vi "_wmg_readItems.vi"(2 "input_p":i32[](array[numeric]), 3 "input":string[](array[string]), 4 "input_sp":string[](array[string])) -> (0 "output_p":i32[](array[numeric]), 1 "output_sp":string[](array[string]))   [LabVIEW 2011]
panel:
  out "数组":string[](array[string])
  in  "列表框":i32(listbox)
  out "数组 2":i32[](array[numeric])
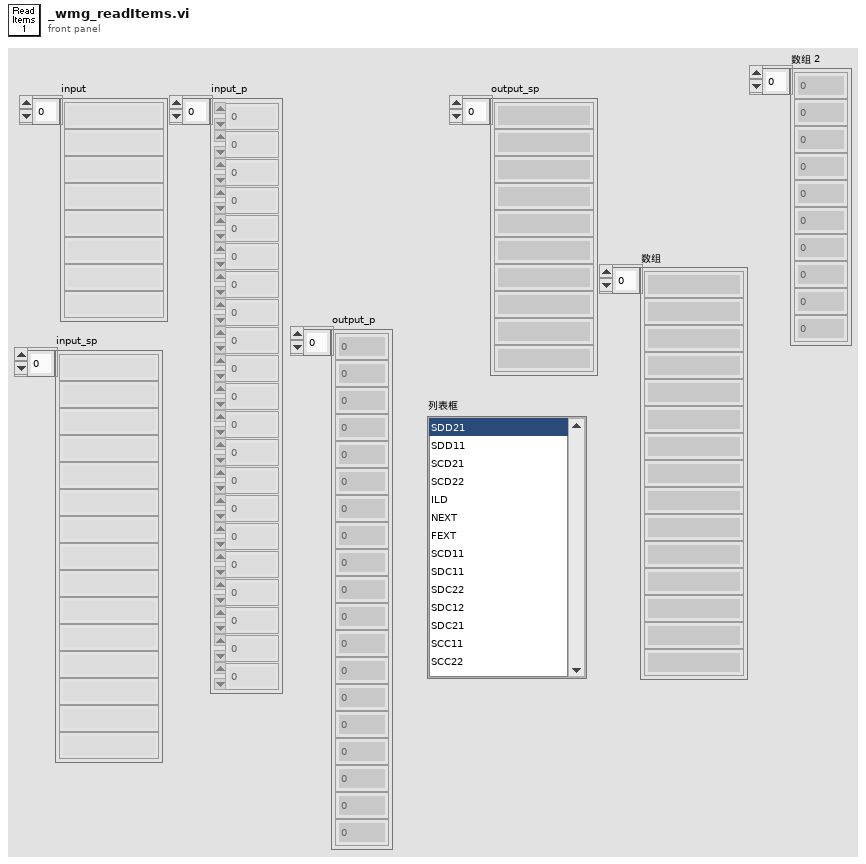
[diagram p1: front panel]
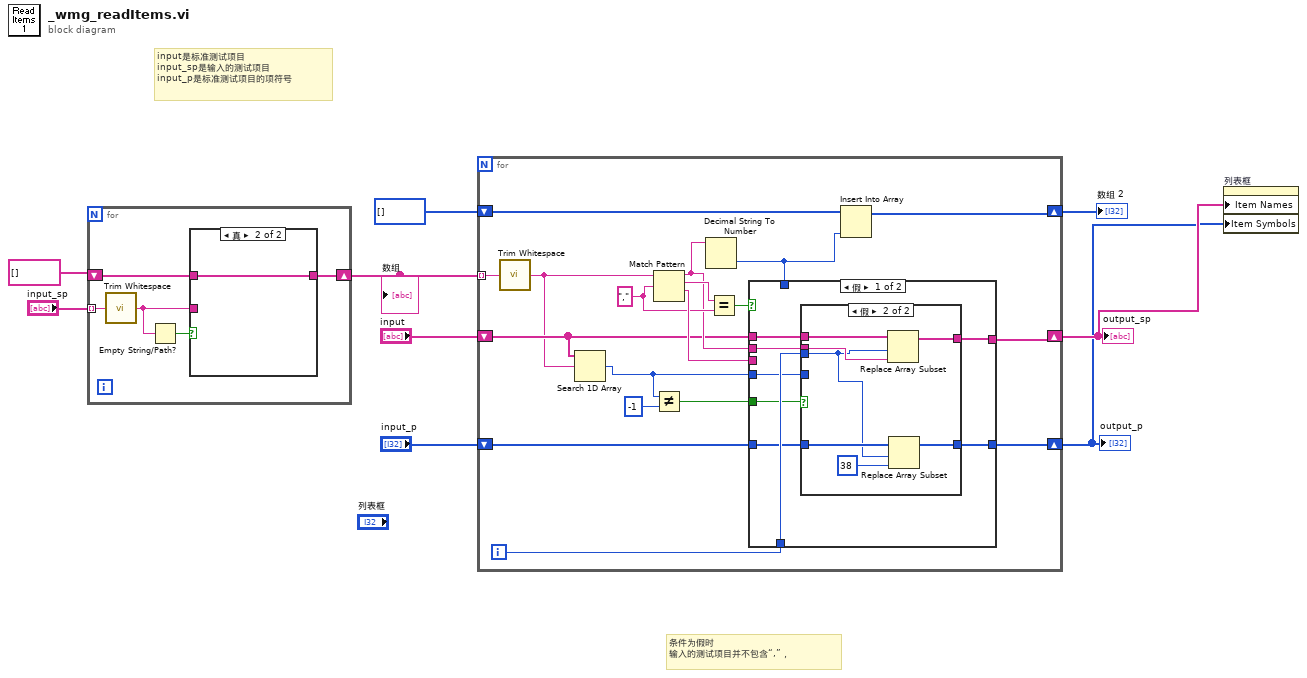
[diagram p0: block diagram]
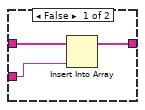
[diagram p2: hidden frame]
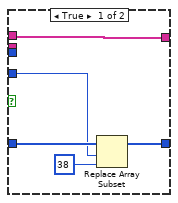
[diagram p3: hidden frame]
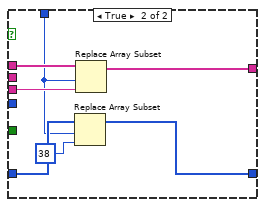
[diagram p4: hidden frame]
diagram:
  # "条件为假时\n输入的测试项目并不包含“,”，"
  # "input是标准测试项目\ninput_sp是输入的测试项目\ninput_p是标准测试项目的项符号"
  n1 = for {
    tunnel: "input_sp" -> [w14] mode=indexing
    shift-right: [w11] -> w5
    shift-left: string[] [] -> [w12]
    n2 = call <vilib>:"Trim Whitespace.vi"("string"=w14) -> ("trimmed string"=w10:string)  [unwired: 1 in]
    n3 = Empty String/Path?(string/path=w10) -> (empty?=w13:bool)
    n4 = case shown="真" w13 {
      tunnel: w12 -> [w17 w18]
      tunnel: [w16 w18] -> w11
      tunnel: w10 -> [w15 _]
      frame False {
        n5 = Insert Into Array(array=w17, new element=w15) -> (w16:string[])  [unwired: 1 in]
      }
      frame True {
      }
    }
  }
  "数组" <- w5
  n6 = for {
    tunnel: w5 -> [w36] mode=indexing
    shift-right: [w34] -> w2
    shift-left: "input" -> [w23]
    shift-right: [w32] -> w1
    shift-left: "input_p" -> [w33]
    shift-right: [w29] -> w3
    shift-left: i32[] [] -> [w31]
    i -> [w24]
    w27 = "," ("正则表达式")
    n7 = call <vilib>:"Trim Whitespace.vi"("string"=w36) -> ("trimmed string"=w22:string)  [unwired: 1 in]
    n8 = Search 1D Array(1D array=w23, element=w22) -> (index of element=w21:i32)  [unwired: 1 in]
    n9 = Match Pattern(string=w22, regular expression=w27) -> (before substring=w25:string, match substring=w28:string, after substring=w35:string)  [unwired: 1 in, 1 out]
    n10 = Not Equal?(x=w21, y=-1) -> (x != y?=w19:bool)
    n11 = Decimal String To Number(string=w25) -> (number=w30:i32)  [unwired: 2 in, 1 out]
    n12 = Equal?(x=w28, y=w27) -> (x = y?=w26:bool)
    n13 = case shown="假" w26 {
      tunnel: w23 -> [w44 w63]
      tunnel: w35 -> [_ w62]
      tunnel: [w43 w61] -> w34
      tunnel: w33 -> [w40 w60]
      tunnel: [w39 w59] -> w32
      tunnel: w30 -> [_ w57]
      tunnel: w25 -> [w42 _]
      tunnel: w24 -> [w41 _]
      tunnel: w21 -> [w38 _]
      tunnel: w19 -> [w37 _]
      frame False {
        n14 = case shown="假" w37 {
          tunnel: w44 -> [w45 w56]
          tunnel: [w45 w55] -> w43
          tunnel: w42 -> [_ w54]
          tunnel: w41 -> [_ w50]
          tunnel: w40 -> [w49 w53]
          tunnel: [w48 w52] -> w39
          tunnel: w38 -> [w47 _]
          frame True {
            n15 = Replace Array Subset(array=w49, new element=38 ("新元素/子数组"), index=w47) -> (w48:i32[])
          }
          frame False {
            n16 = Replace Array Subset(array=w56, new element=w54, index=w50) -> (w55:string[])
            n17 = Replace Array Subset(array=w53, new element=38 ("新元素/子数组"), index=w50) -> (w52:i32[])
          }
        }
      }
      frame True {
        n18 = Replace Array Subset(array=w60, new element=38 ("新元素/子数组"), index=w57) -> (w59:i32[])
        n19 = Replace Array Subset(array=w63, new element=w62, index=w57) -> (w61:string[])
      }
    }
    n20 = Insert Into Array(array=w31, new element=w30) -> (w29:i32[])  [unwired: 1 in]
  }
  "output_sp" <- w2
  "output_p" <- w1
  "数组 2" <- w3
  n21 = property on="列表框" class="LstBox (严格)"("Item Names"=w2, "Item Symbols"=w1) -> ()  [unwired: 2 in, 2 out]
